vi "AlliGator Rescale 2-Exp Fraction.vi"(9 "2-Exp Parameters":T1, 11 "a 1 in":dbl) -> (3 "r 1 out":dbl)   [LabVIEW 2021, in "AlliGator Fit Method Benchmark.lvlib"]
doc: "Normalizes decay amplitudes for random timestamp generation."
uses:
  AlliGator Fit Method Benchmark.lvlib
  AlliGator 2-Exp Parameters.ctl
panel:
  # "see the AlliGator License on the block diagram (Ctrl+E or Window:Show Block Diagram)"
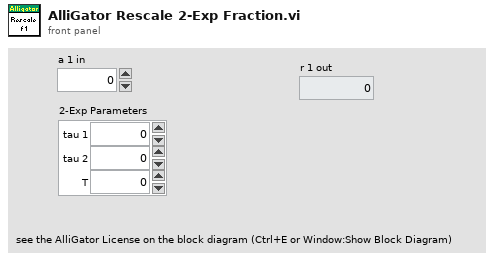
[diagram p1: front panel]
types:
  T1 = typedef "AlliGator Fit Method Benchmark.lvlib/AlliGator 2-Exp Parameters.ctl" = cluster{"tau 1":dbl, "tau 2":dbl, "T":dbl}
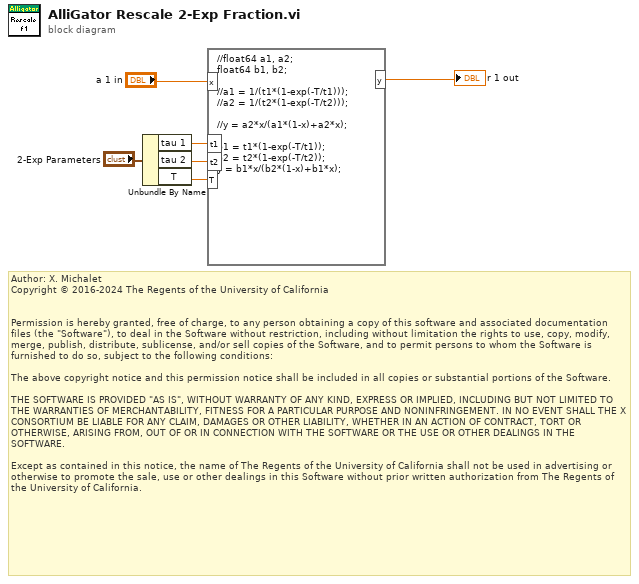
[diagram p0: block diagram]
diagram:
  # "Author: X. Michalet\nCopyright © 2016-2024 The Regents of the University of California\n \n\nPermission is hereby granted, free of charge, to any person obtaining a copy of this software and associated documentation files (the \"Software\"), to deal in the Software without restriction, including without limitation the rights to use, copy, modify, merge, publish, distribute, sublicense, and/or sell copies of the Software, and to permit persons to whom the Software is furnished to do so, subject to the following conditions:\n\nThe above copyright notice and this permission notice shall be included in all copies or substantial portions of the Software.\n\nTHE SOFTWARE IS PROVIDED \"AS IS\", WITHOUT WARRANTY OF ANY KIND, EXPRESS OR IMPLIED, INCLUDING BUT NOT LIMITED TO THE WARRANTIES OF MERCHANTABILITY, FITNESS FOR A PARTICULAR PURPOSE AND NONINFRINGEMENT. IN NO EVENT SHALL THE X CONSORTIUM BE LIABLE FOR ANY CLAIM, DAMAGES OR OTHER LIABILITY, WHETHER IN AN ACTION OF CONTRACT, TORT OR OTHERWISE, ARISING FROM, OUT OF OR IN CONNECTION WITH THE SOFTWARE OR THE USE OR OTHER DEALINGS IN THE SOFTWARE.\n\nExcept as contained in this notice, the name of The Regents of the University of California shall not be used in advertising or otherwise to promote the sale, use or other dealings in this Software without prior written authorization from The Regents of the University of California."
  n1 = Unbundle By Name("2-Exp Parameters") -> ("tau 1"=w3:dbl, "tau 2"=w2:dbl, "T"=w1:dbl)
  n2 = formula code="//float64 a1, a2;\nfloat64 b1, b2;\n\n//a1 = 1/(t1*(1-exp(-T/t1)));\n//a2 = 1/(t2*(1-exp(-T/t2)));\n\n//y = a2*x/(a1*(1-x)+a2*x);\n\nb1 = t1*(1-exp(-T/t1));\nb2 = t2*(1-exp(-T/t2));\ny = b1*x/(b2*(1-x)+b1*x);"("x"="a 1 in", "t1"=w3, "t2"=w2, "T"=w1) -> ("y"=→"r 1 out":dbl)
